vi "throw with message.vi"(5 "call chain?":bool, 7 "source":string, 8 "exception in":T1 {"code" format="%.0x"}, 9 "message":string, 10 "severity":T3, 11 "code":i32) -> (0 "exception out":T1 {"code" format="%.0x"})   [LabVIEW 2013, in "exception.lvlib"]
uses:
  exception.lvlib
  exception.ctl
  context.ctl
  severity.ctl
  const severityname.vi
  const sourcename.vi
  const messagename.vi
  const exceptioncausename.vi
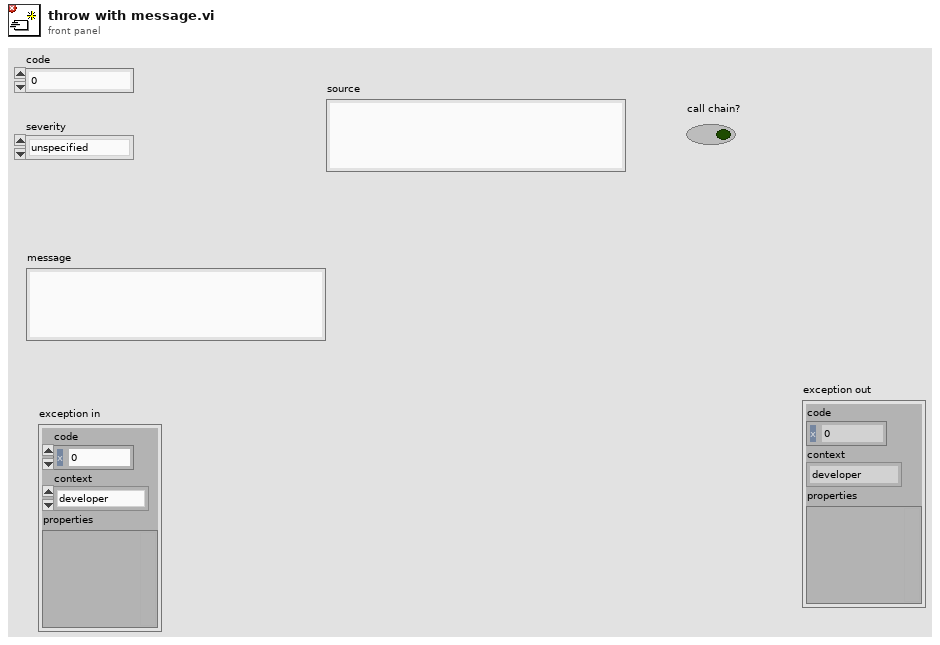
[diagram p1: front panel]
types:
  T1 = typedef "exception.lvlib/exception.ctl" = cluster{"code":i32, "context":T2, "properties":variant}
  T2 = typedef "exception.lvlib/context.ctl" = enum16{"developer", "user interface", "standard", "limited", "deterministic"}
  T3 = typedef "exception.lvlib/severity.ctl" = enum8{"unspecified", "operation failed", "data corruption", "system corruption", "critical unknown state"}
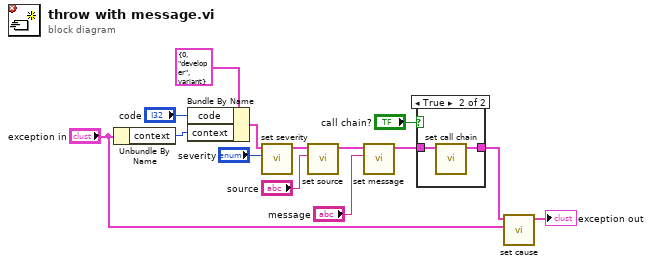
[diagram p0: block diagram]
diagram:
  n1 = Unbundle By Name("exception in") -> ("context"=w1:T2)
  n2 = Bundle By Name(cluster=T1 {"code"=0, "context"=enum."developer", "properties"=variant} ("exception"), "code"="code", "context"=w1) -> (w13:T1)
  n3 = call "set severity.vi"("severity"="severity", "exception in"=w13) -> ("exception out"=w5:T1)  [unwired: 9 in]
  n4 = call "set source.vi"("source"="source", "exception in"=w5) -> ("exception out"=w11:T1)  [unwired: 9 in]
  n5 = call "set message.vi"("message"="message", "exception in"=w11) -> ("exception out"=w9:T1)  [unwired: 9 in]
  n6 = case shown="True" "call chain?" {
    tunnel: w9 -> [w15 w17]
    tunnel: [w15 w16] -> w6
    frame False {
    }
    frame True {
      n7 = call "set call chain.vi"("exception in"=w17) -> ("exception out"=w16:T1)  [unwired: 10 in]
    }
  }
  n8 = call "set cause.vi"("cause"="exception in", "exception in"=w6) -> ("exception out"=→"exception out":T1)  [unwired: 9 in]
